vi "Parse Signal List.vi"(8 "error in (no error)":errorcluster, 9 "Signal List":string[][](array[string]), 10 "Headers":string[](array[string]), 11 "Relay Names":string[](array[string])) -> (0 "error out":errorcluster, 1 "Names":string[](array[string]))   [LabVIEW 2019]
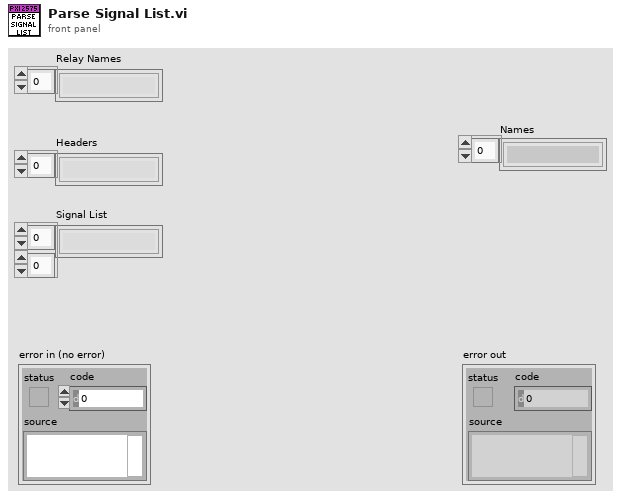
[diagram p1: front panel]
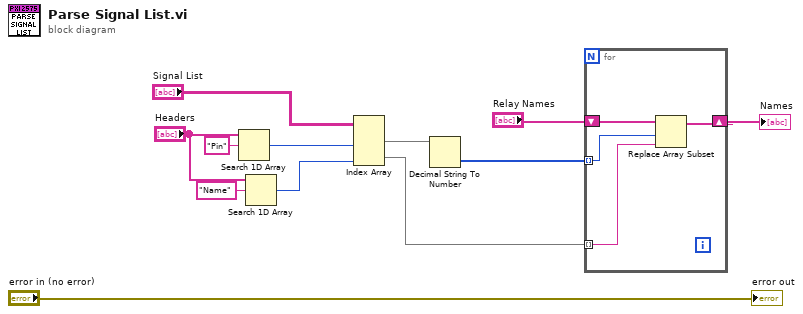
[diagram p0: block diagram]
diagram:
  n1 = Search 1D Array(1D array="Headers", element="Pin") -> (index of element=w8:i32)  [unwired: 1 in]
  n2 = Search 1D Array(1D array="Headers", element="Name") -> (index of element=w11:i32)  [unwired: 1 in]
  n3 = Index Array(array="Signal List", index (col) #1=w8, index (col) #2=w11) -> (element #1=w9:string[], element #2=w3:string[])  [unwired: 2 in]
  n4 = Decimal String To Number(string=w9) -> (number=w4:i32[])  [unwired: 2 in, 1 out]
  n5 = for {
    tunnel: w4 -> [w13] mode=indexing
    tunnel: w3 -> [w14] mode=indexing
    shift-right: [w15] -> w2
    shift-left: "Relay Names" -> [w16]
    n6 = Replace Array Subset(array=w16, new element=w14, index=w13) -> (w15:string[])
  }
  "Names" <- w2
  "error out" <- "error in (no error)"
